vi "Start Sync.vi"(8 "error in (no error)":errorcluster, 11 "gRPC Server in":refnum<class "ServiceManagementService.lvclass">) -> (0 "error out":errorcluster, 3 "gRPC Server out":refnum<class "ServiceManagementService.lvclass">)   [LabVIEW 2020, in "LineRegulation.lvlib" / "ServiceManagementService.lvclass"]
uses:
  ServiceManagementService.lvclass
  ServiceManagementService.lvclass/ServiceManagementService.ctl
  RPC Messages/ni_measurements_servicemanagement_v1_StopServiceResponse.ctl
  LineRegulation.lvlib
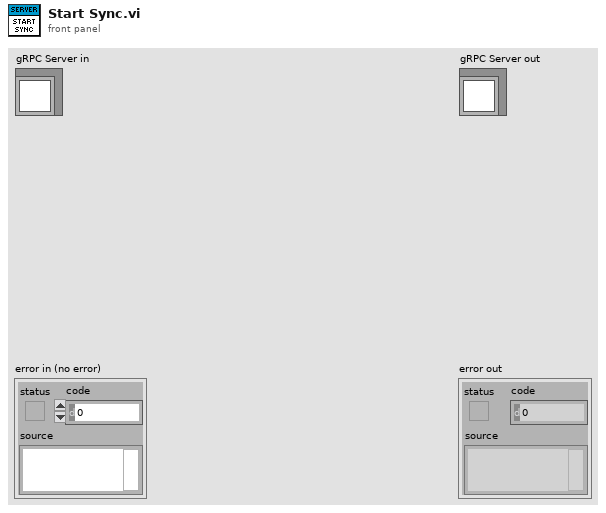
[diagram p1: front panel]
types:
  T1 = typedef "LineRegulation.lvlib/ni_measurements_servicemanagement_v1_StopServiceResponse.ctl" = cluster{"void":string}
  T2 = typedef "LineRegulation.lvlib/ServiceManagementService.lvclass/Server Internal UEs.ctl" = cluster{"ni_servicemanagement_v1_ServiceManagementService_StopService Internal UE":refnum<user-event>, "ni_measurements_servicemanagement_v1_ServiceManagementService_StopService Internal UE":refnum<user-event>}
  T3 = typedef "LineRegulation.lvlib/ServiceManagementService.lvclass/Server gRPC UEs.ctl" = cluster{"ni_servicemanagement_v1_ServiceManagementService_StopService gRPC UE":refnum<user-event>, "ni_measurements_servicemanagement_v1_ServiceManagementService_StopService gRPC UE":refnum<user-event>}
  T4 = typedef "gprc-lvsupport-release.lvlib/grpcId.ctl" = u64
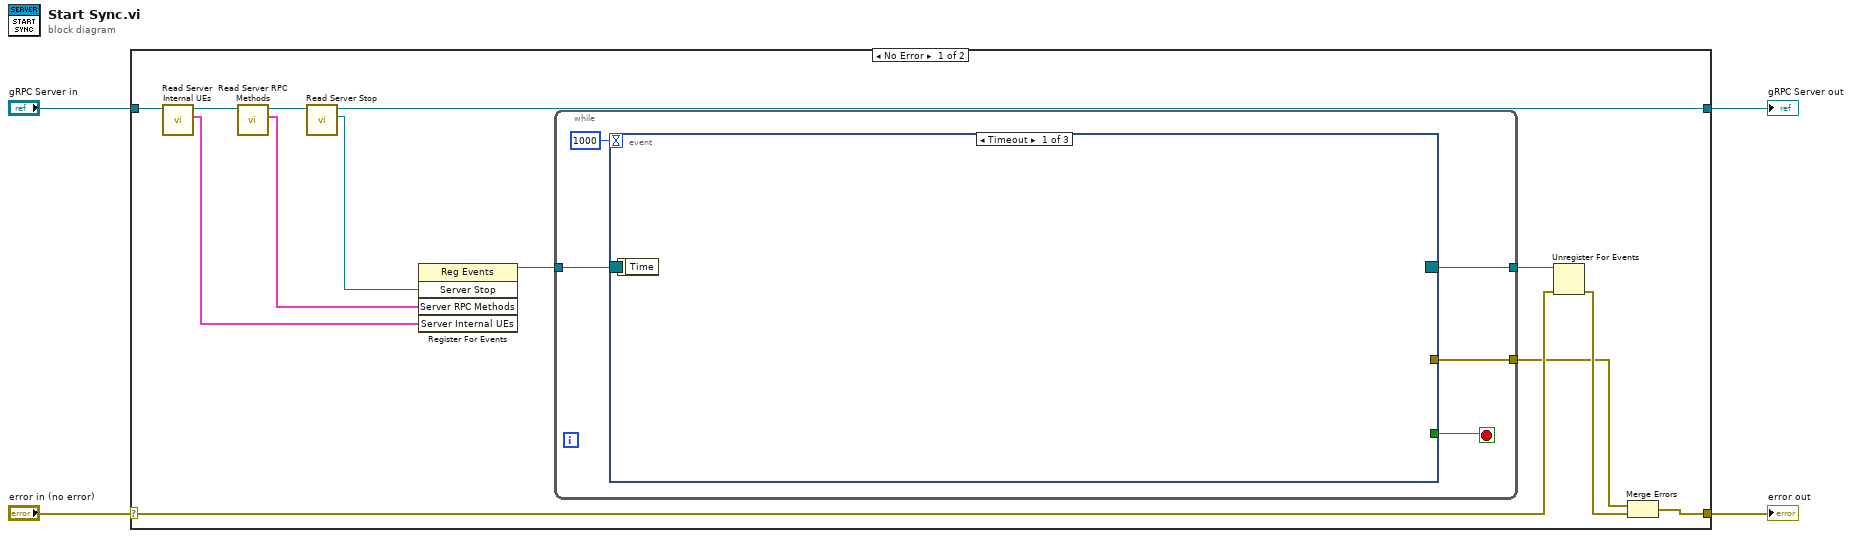
[diagram p0: block diagram]
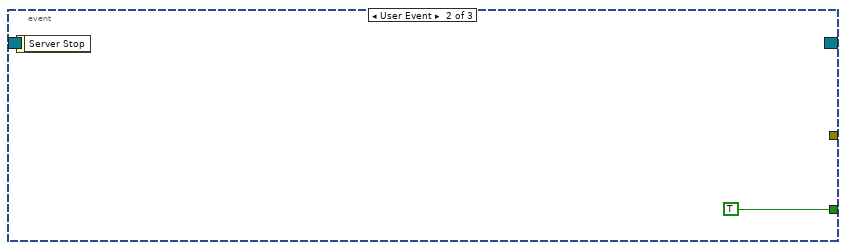
[diagram p2: hidden frame]
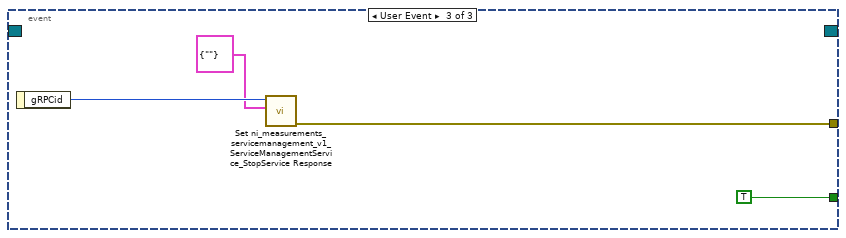
[diagram p3: hidden frame]
diagram:
  n1 = case shown="No Error" "error in (no error)" {
    selector: "error in (no error)" -> [w11 w29]
    tunnel: [w6 w29] -> w3
    tunnel: [w8 w28] -> w1
    tunnel: "gRPC Server in" -> [w17 w28]
    frame No Error {
      n2 = call "Read Server Internal UEs.vi"("SignalGeneratorService in"=w17) -> ("Server Internal UEs"=w15:T2, "SignalGeneratorService out"=w16:refnum<class "ServiceManagementService.lvclass">)  [unwired: 8 in, 1 out]
      n3 = call "Read Server RPC Methods.vi"("SignalGeneratorService in"=w16) -> ("Server RPC Methods"=w9:T3, "SignalGeneratorService out"=w14:refnum<class "ServiceManagementService.lvclass">)  [unwired: 8 in, 1 out]
      n4 = call-dynamic "Read Server Stop.vi"("iService in"=w14) -> ("Server Stop"=w7:refnum<user-event>, "iService out"=w8:refnum<class "ServiceManagementService.lvclass">)  [unwired: 8 in, 1 out]
      n5 = register-events(w7, w9, w15) -> (reference out=w13:refnum<event-registration>)  [unwired: 2 in, 1 out]
      n6 = while {
        tunnel: w13 -> [w22]
        tunnel: [w20] -> w12
        tunnel: [w18] -> w5
        stop <- w21 stop-if-true
        n7 = event "RPC Methods Event Structure" shown="[0] Timeout" {
          selector: w22 -> [_ _ _]
          dyn-events: [_ _ _] -> w20
          timeout: 1000 -> [_ _ _]
          tunnel: [_ TRUE TRUE] -> w21
          tunnel: [_ _ w25] -> w18
          event Timeout {
            n8 = event-data() -> ()  [unwired: 1 in, 1 out]
          }
          event User Event {
            n9 = event-data() -> ()  [unwired: 1 in, 1 out]
          }
          event User Event {
            n10 = event-data() -> ("gRPCid"=w26:T4)  [unwired: 1 in]
            n11 = call "Set ni_measurements_servicemanagement_v1_ServiceManagementService_StopService Response.vi"("Message Data"=T1 {"void"=""}, "gRPCid in"=w26) -> ("error out"=w25:errorcluster)  [unwired: 9 in]
          }
        }
      }
      n12 = Unregister For Events(event registration refnum=w12, error in=w11) -> (error out=w10:errorcluster)
      n13 = Merge Errors(w5, w10) -> (w6:errorcluster)
    }
    frame Error {
    }
  }
  "error out" <- w3
  "gRPC Server out" <- w1
